vi "test single REQ v2.vi"() -> ()   [LabVIEW 2018, in "LV-0mq-Julia_roundtrip-lib.lvlib"]
uses:
  LV-0mq-Julia_roundtrip-lib.lvlib
  Commands.ctl
  commands LV2Jl.ctl
  <vilib>/addons/zeromq/zmq_socket.lvclass
panel:
  in  "use binary data":bool
  in  "binary data in":u8[](array[numeric])=[1, 2, 3, 4]
  in  "JSON data in":string="{\"fun2call\":\"myf1\", \"arg1\":0, \"arg2\":3.1415}"
  in  "Command":T1=99 items=["call function"=99, "ping"=112, "stop"=115, "unused"=254]
  out "short err code":u8
  out "roundtrip time":dbl
  out "detailed err description":string
  out "JSON data":string
  out "binary data out":u8[](array[numeric])
  out "server response":string
  out "error out":errorcluster
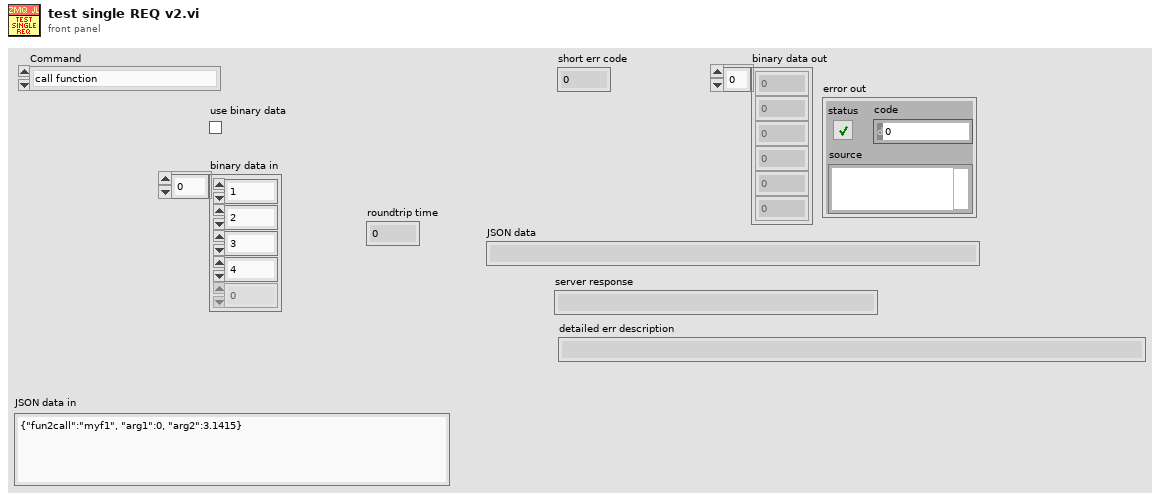
[diagram p1: front panel]
types:
  T1 = typedef "LV-0mq-Julia_roundtrip-lib.lvlib/commands LV2Jl.ctl" = u8
  T2 = typedef "LV-0mq-Julia_roundtrip-lib.lvlib/Commands.ctl" = enum16{"Start Jl-server & Init LV-client", "Send request & Get response ", "Stop Jl-server & Cleanup LV-client", "Cleanup LV-client", "Start Jl-server", "Stop Jl-server", "Init LV-Client", "Cleanup LV-Client", "(not allowed)", "Set LV Client state", "Set Jl Server state", "set ZMQ timeout", "read ZMQ timeout", "read-out state"}
  T3 = typedef "LV-0mq-Julia_roundtrip-lib.lvlib/detailed error info.ctl" = cluster{"exception_or_info":string, "trace":T4[]}
  T4 = typedef "LV-0mq-Julia_roundtrip-lib.lvlib/StackFrame.ctl" = cluster{"frame_summary":string, "func":string, "linfo":string, "file":string, "line":i32, "pointer":u64, "from_c":bool, "inlined":bool}
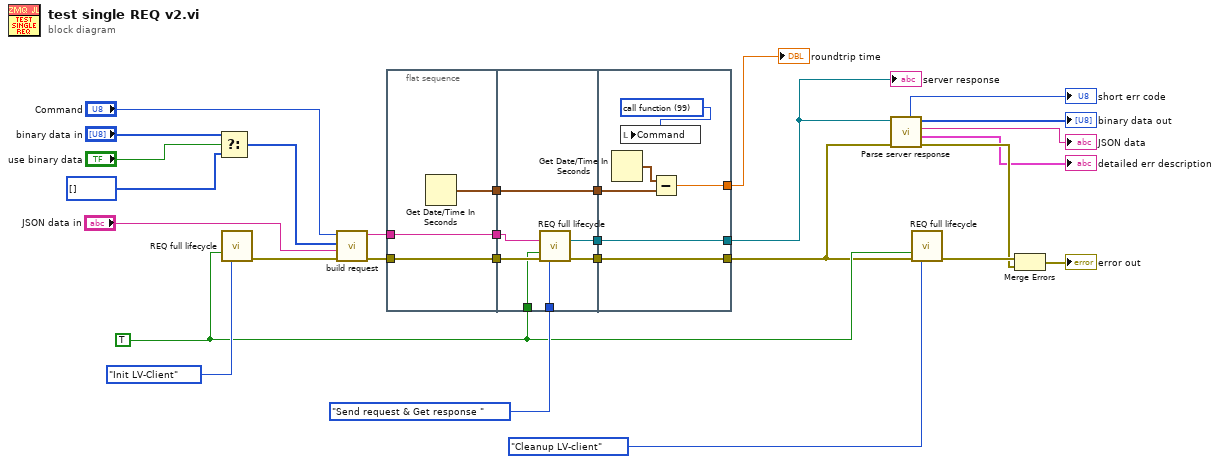
[diagram p0: block diagram]
diagram:
  w25 = TRUE ("Force command")
  n1 = Select(t="binary data in", s="use binary data", f=u8[] [] ("binary data in 2")) -> (s? t:f=w2:u8[])
  n2 = call "REQ full lifecycle.vi"("Force command"=w25, "command"=Commands."Init LV-Client") -> ("error out"=w10:errorcluster)  [unwired: 7 in, 6 out]
  n3 = call "build request.vi"("error in (no error)"=w10, "JSON data"="JSON data in", "binary data"=w2, "Command"="Command") -> ("error out"=w9:errorcluster, "REQ string"=w7:string)  [unwired: 6 in]
  n4 = flat-sequence {
    tunnel: w9 -> [w32]
    tunnel: [w32] -> w15
    tunnel: [w31] -> w14
    tunnel: [w30] -> w8
    tunnel: w7 -> [w30]
    tunnel: Commands."Send request & Get response " ("command") -> [w38]
    tunnel: w25 -> [w37]
    tunnel: [w36] -> w17
    tunnel: [w35] -> w16
    tunnel: w15 -> [w39]
    tunnel: w14 -> [w34]
    tunnel: [w34] -> w13
    tunnel: w8 -> [w33]
    tunnel: [w44] -> w23
    tunnel: [w45] -> w24
    tunnel: w17 -> [w45]
    tunnel: w16 -> [w44]
    tunnel: w13 -> [w42]
    tunnel: [w41] -> w12
    frame #0 {
      n5 = Get Date/Time In Seconds() -> (seconds since 1Jan1904=w31:timestamp)
    }
    frame #1 {
      n6 = call "REQ full lifecycle.vi"("data to send"=w33, "Force command"=w37, "error in"=w39, "command"=w38) -> ("socket out"=w36:refnum<class "zmq_socket.lvclass">, "error out"=w35:errorcluster)  [unwired: 5 in, 5 out]
    }
    frame #2 {
      w40 = T1 99 items=["call function"=99, "stop"=112] ("Command")
      n7 = Get Date/Time In Seconds() -> (seconds since 1Jan1904=w43:timestamp)
      n8 = local write "Command"(w40) -> ()
      n9 = Subtract(x=w43, y=w42) -> (x-y=w41:dbl)
    }
  }
  n10 = call "Parse server response.vi"("error in (no error)"=w23, "server response in"=w24) -> ("error out"=w21:errorcluster, "detailed error info"=→"detailed err description":T3, "JSON out"=→"JSON data":string, "binary data"=→"binary data out":u8[], "return code"=→"short err code":u8)  [unwired: 2 in, 3 out]
  n11 = call "REQ full lifecycle.vi"("Force command"=w25, "error in"=w23, "command"=Commands."Cleanup LV-client") -> ("error out"=w27:errorcluster)  [unwired: 6 in, 6 out]
  n12 = Merge Errors(w27, w21) -> (→"error out":errorcluster)
  "server response" <- w24
  "roundtrip time" <- w12
